vi "VariableManager_String.vi"(7 "Operation":enum16{"Get Tag", "Set Tag"}(ring), 8 "error in (no error)":errorcluster, 10 "Value":string, 11 "Tag":string) -> (0 "error out":errorcluster, 2 "Value out":string, 3 "Tag Out":string, 4 "Found":bool)   [LabVIEW 2021]
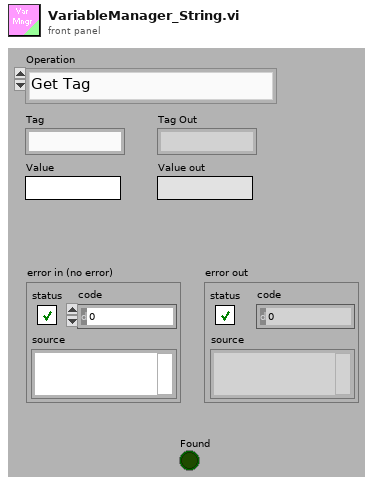
[diagram p1: front panel]
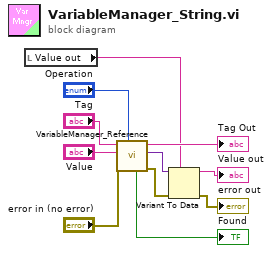
[diagram p0: block diagram]
diagram:
  n1 = local read "Value out"() -> (w1:string)
  n2 = call "VariableManager_Reference.vi"("Operation"="Operation", "error in (no error)"="error in (no error)", "Value"="Value", "Tag"="Tag") -> ("error out"=w6:errorcluster, "Value out"=w7:variant, "Tag Out"=→"Tag Out":string, "Found"=→"Found":bool)  [unwired: 3 in, 1 out]
  n3 = Variant To Data(error in=w6, type=w1, Variant=w7) -> (data=→"Value out":string, error out=→"error out":errorcluster)
